vi "Skate.vi"(2 "Power":i32 max=100 step=1, 3 "BrickReference in":T1) -> (1 "BrickReference out":T1)   [LabVIEW 2015]
uses:
  <vilib>/NXT/Subs/LVHSConnector.ctl
  <vilib>/NXT/LegoClasses/BrickReference/BrickReference.lvclass
  <vilib>/NXT/Subs/MotorOutput.ctl
  <vilib>/NXT/Block Support/NXT_TimerIndex.ctl
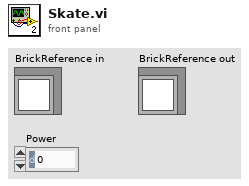
[diagram p1: front panel]
types:
  T1 = typedef "LVHSConnector.ctl" = refnum<class "BrickReference.lvclass">
  T2 = typedef "NXT_TimerIndex.ctl" = u8
  T3 = typedef "MotorOutput.ctl" = u8
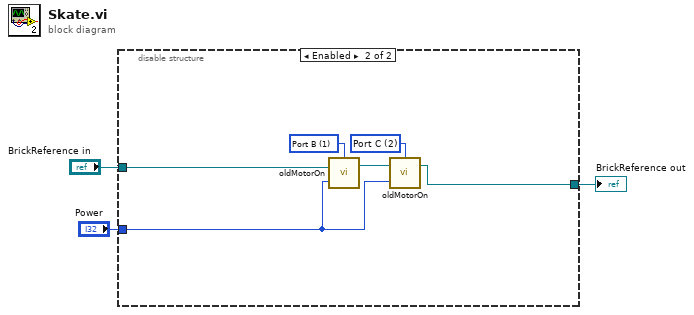
[diagram p0: block diagram]
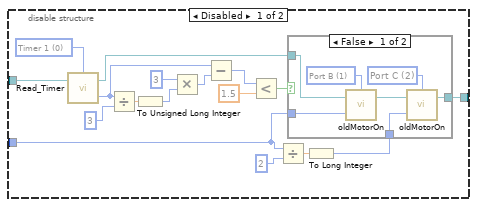
[diagram p2: hidden frame]
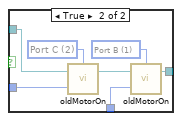
[diagram p3: hidden frame]
diagram:
  n1 = disable-structure shown="Enabled" {
    disable-tunnel: "BrickReference in" -> [w7 w40]
    disable-tunnel: [w6 w36] -> w2
    disable-tunnel: "Power" -> [w5 w35]
    frame Disabled {
      w19 = T2 0 items=["Timer 1", "Timer 2", "Timer 3"] ("Timer (Timer 1)")
      n2 = call <vilib>:"Read_Timer.vi"("NXT/EV3"=w7, "Timer (Timer 1)"=w19) -> ("Value (msec)"=w16:u32, "NXT/EV3"=w4:T1)  [unwired: 1 in]
      n3 = Divide(x=w16, y=u32 3) -> (x/y=w17:dbl)
      n4 = To Unsigned Long Integer(number=w17) -> (unsigned 32bit integer=w15:u32)
      n5 = Multiply(x=u32 3, y=w15) -> (x*y=w13:u32)
      n6 = Subtract(x=w16, y=w13) -> (x-y=w12:u32)
      n7 = Less?(x=w12, y=1.5) -> (x < y?=w8:bool)
      n8 = Divide(x=w5, y=u8 2) -> (x/y=w10:dbl)
      n9 = To Long Integer(number=w10) -> (32bit integer=w11:i32)
      n10 = case shown="False" w8 {
        tunnel: w5 -> [w23 w30]
        tunnel: [w24 w31] -> w6
        tunnel: w11 -> [w22 w29]
        tunnel: w4 -> [w21 w28]
        frame False {
          w26 = T3 2 items=["Port A"=0, "Port B"=1, "Port C"=2, "Ports A & B"=4, "Ports A & C"=5, "Ports B & C"=6, "All Ports"=3] ("Output Port (All Ports)")
          w25 = T3 1 items=["Port A"=0, "Port B"=1, "Port C"=2, "Ports A & B"=4, "Ports A & C"=5, "Ports B & C"=6, "All Ports"=3] ("Output Port (All Ports)")
          n11 = call <vilib>:"oldMotorOn.vi"("Power (75)"=w23, "NXT/EV3"=w21, "Output Port (All Ports)"=w25) -> ("NXT/EV3"=w27:T1)  [unwired: 1 in]
          n12 = call <vilib>:"oldMotorOn.vi"("Power (75)"=w22, "NXT/EV3"=w27, "Output Port (All Ports)"=w26) -> ("NXT/EV3"=w24:T1)  [unwired: 1 in]
        }
        frame True {
          w33 = T3 1 items=["Port A"=0, "Port B"=1, "Port C"=2, "Ports A & B"=4, "Ports A & C"=5, "Ports B & C"=6, "All Ports"=3] ("Output Port (All Ports)")
          w32 = T3 2 items=["Port A"=0, "Port B"=1, "Port C"=2, "Ports A & B"=4, "Ports A & C"=5, "Ports B & C"=6, "All Ports"=3] ("Output Port (All Ports)")
          n13 = call <vilib>:"oldMotorOn.vi"("Power (75)"=w30, "NXT/EV3"=w28, "Output Port (All Ports)"=w32) -> ("NXT/EV3"=w34:T1)  [unwired: 1 in]
          n14 = call <vilib>:"oldMotorOn.vi"("Power (75)"=w29, "NXT/EV3"=w34, "Output Port (All Ports)"=w33) -> ("NXT/EV3"=w31:T1)  [unwired: 1 in]
        }
      }
    }
    frame Enabled {
      w38 = T3 2 items=["Port A"=0, "Port B"=1, "Port C"=2, "Ports A & B"=4, "Ports A & C"=5, "Ports B & C"=6, "All Ports"=3] ("Output Port (All Ports)")
      w37 = T3 1 items=["Port A"=0, "Port B"=1, "Port C"=2, "Ports A & B"=4, "Ports A & C"=5, "Ports B & C"=6, "All Ports"=3] ("Output Port (All Ports)")
      n15 = call <vilib>:"oldMotorOn.vi"("Power (75)"=w35, "NXT/EV3"=w40, "Output Port (All Ports)"=w37) -> ("NXT/EV3"=w39:T1)  [unwired: 1 in]
      n16 = call <vilib>:"oldMotorOn.vi"("Power (75)"=w35, "NXT/EV3"=w39, "Output Port (All Ports)"=w38) -> ("NXT/EV3"=w36:T1)  [unwired: 1 in]
    }
  }
  "BrickReference out" <- w2
